vi "IRH1-2T_ConstructiveHeuristic.vi"(9 "Initial Construction Heursitic":T2, 10 "Scheduler":T1, 11 "Proocessing Times MxJ":u16[][](array[numeric])=[[1, 69, 192, 47, 292, 28, 166, 205], [146, 96, 177, 62, 37, 145, 3, 334], [99, 182, 133, 113, 9, 239, 27, 198], [159, 182, 132, 158, 183, 38, 142, 6], [92, 63, 114, 144, 180, 199, 136, 72], [119, 31, 9, 163, 139, 158, 350, 31], [46, 30, 59, 290, 156, 90, 175, 154], [338, 347, 184, 23, 4, 103, 1, 0]]) -> (1 "Due Dates":u16[](array[numeric]), 2 "Total Tardiness":u16, 3 "IRH2T Schedule Out":u16[](array[numeric]))   [LabVIEW 2013]
uses:
  Initial Construction Heuristic.ctl
  GA/Controls/Scheduler Type.ctl
  Classes/Scheduler_Class/Prins FIFO Scheduler Methods and Controls/Methods/UpdateMachineGaps.vi
  Classes/Scheduler_Class/Prins FIFO Scheduler Methods and Controls/Methods/UpdateJobGaps.vi
  Classes/Scheduler_Class/Prins FIFO Scheduler Methods and Controls/Methods/Find Intersecting Gaps.vi
  Classes/Scheduler_Class/Prins FIFO Scheduler Methods and Controls/Methods/Transform to Plain Job and Machine Gaps Array.vi
  Classes/Scheduler.lvclass
panel:
  in  "Proocessing Times (8x8)":u16[][](array[numeric])=[[1, 69, 192, 47, 292, 28, 166, 205], [146, 96, 177, 62, 37, 145, 3, 334], [99, 182, 133, 113, 9, 239, 27, 198], [159, 182, 132, 158, 183, 38, 142, 6], [92, 63, 114, 144, 180, 199, 136, 72], [119, 31, 9, 163, 139, 158, 350, 31], [46, 30, 59, 290, 156, 90, 175, 154], [338, 347, 184, 23, 4, 103, 1, 0]]
  out "Machine Completion Times":u16[](array[numeric])
  out "Completion Times":u16[][](array[numeric])
  out "Job Completion Times":i32[](array[numeric])
  out "String":string
  out "LPT Array":i32[](array[numeric])
  # "1, 69, 192, 47, 292, 28, 166, 205], \n[146, 96, 177, 62, 37, 145, 3, 334], \n[99, 182, 133, 113, 9, 239, 27, 198], \n[159, 182, 132, 158, 183, 38, 142, 6], \n[92, 63, 114, 144, 180, 199, 136, 72], \n[119, 31, 9, 163, 139, 158, 350, 31], \n[46, 30, 59, 290, 156, 90, 175, 154], \n[338, 347, 184, 23, 4, 103, 1, 0]]"
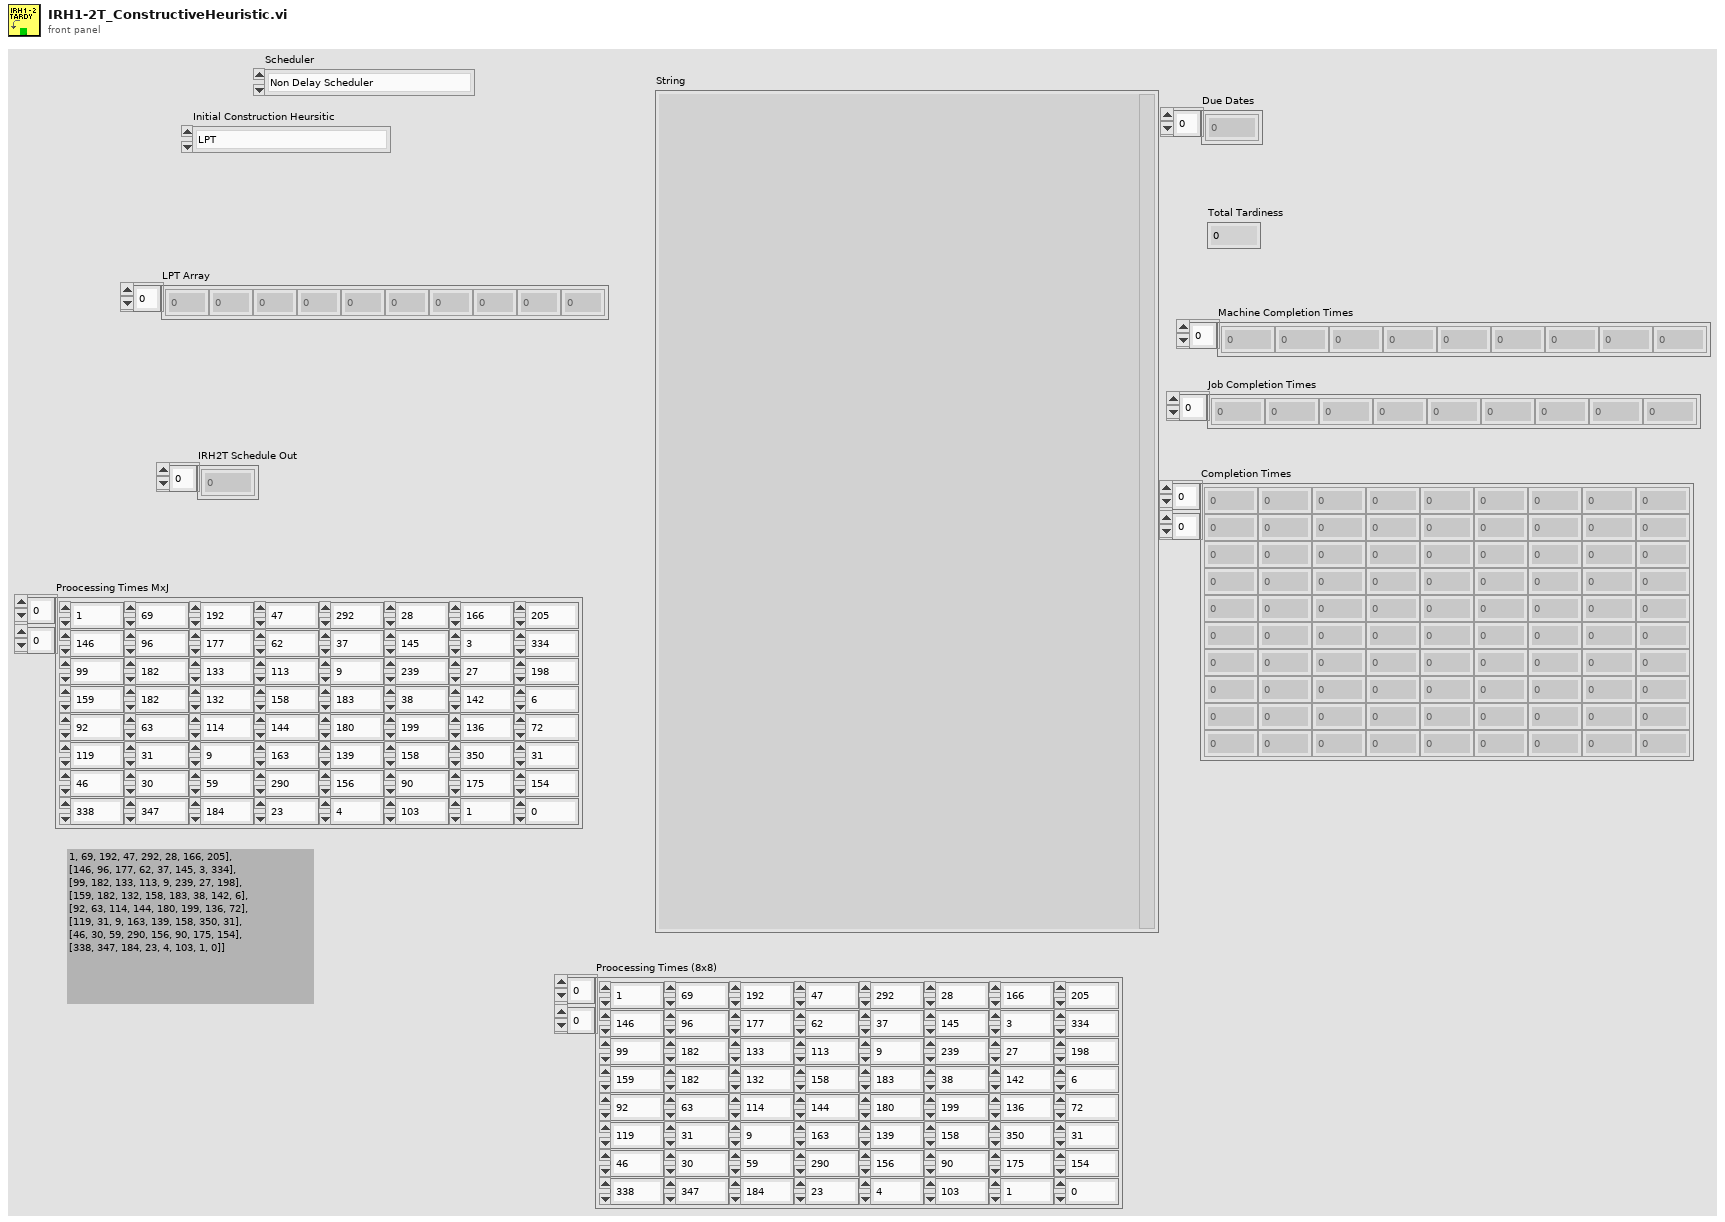
[diagram p1: front panel]
types:
  T1 = typedef "Scheduler Type.ctl" = enum16{"Non Delay Scheduler", "GT Active Scheduler", "My Faulty Scheduler", "Prins FIFO Scheduler", "SemiActive Scheduler", "Modified GT Scheduler"}
  T2 = typedef "Initial Construction Heuristic.ctl" = enum16{"LPT", "SPT", "EDD"}
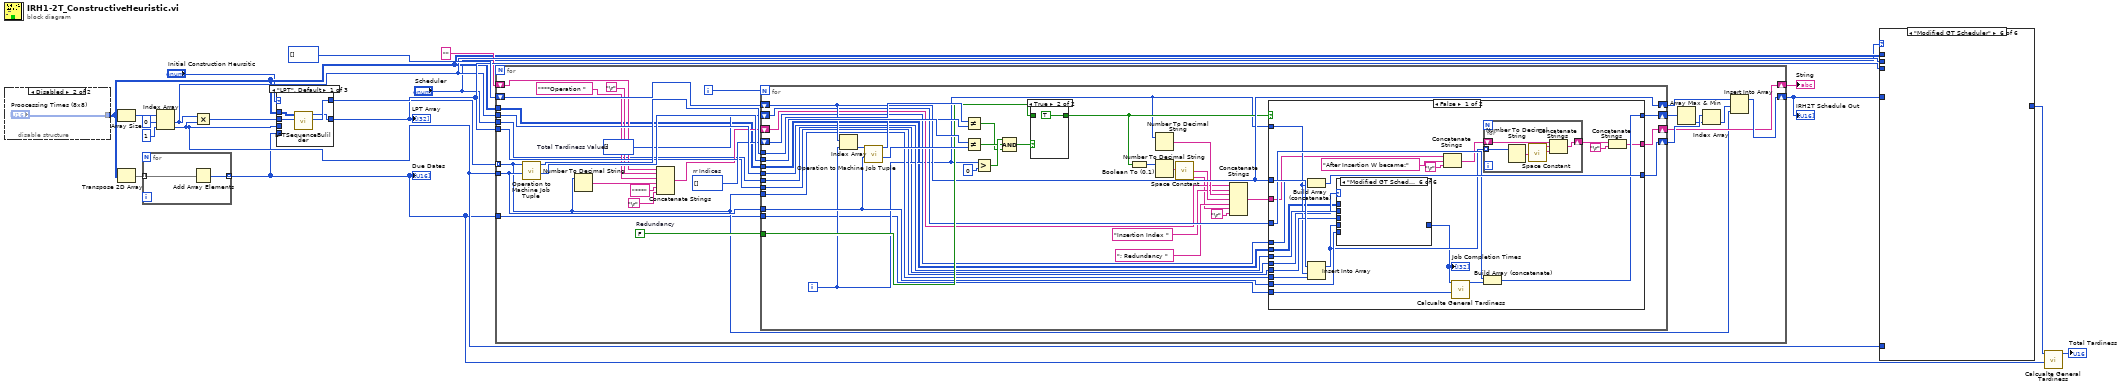
[diagram p0: block diagram]
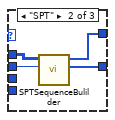
[diagram p2: hidden frame]
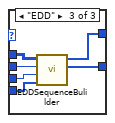
[diagram p3: hidden frame]
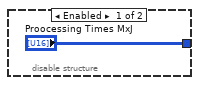
[diagram p4: hidden frame]
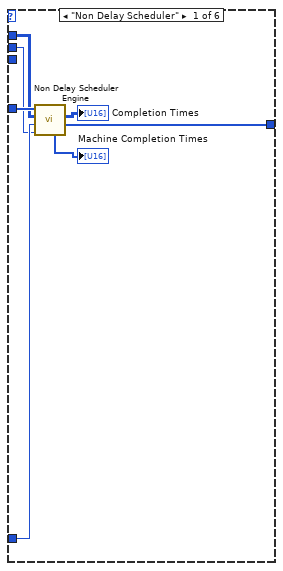
[diagram p5: hidden frame]
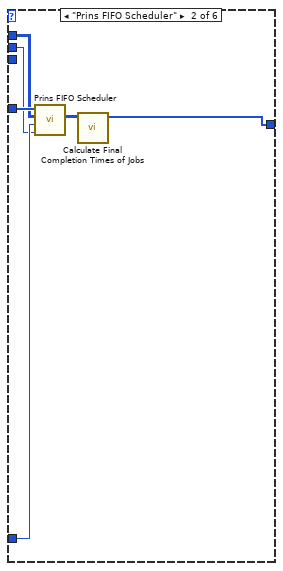
[diagram p6: hidden frame]
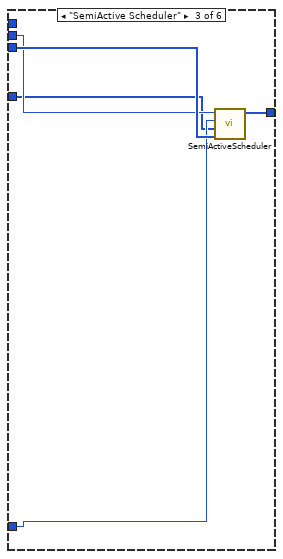
[diagram p7: hidden frame]
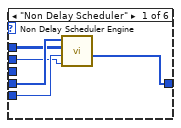
[diagram p10: hidden frame]
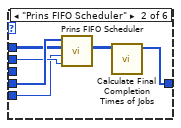
[diagram p11: hidden frame]
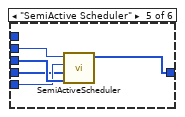
[diagram p14: hidden frame]
diagram:
  n1 = disable-structure shown="Disabled" {
    disable-tunnel: ["Proocessing Times MxJ" "Proocessing Times (8x8)"] -> w7
    frame Enabled {
    }
    frame Disabled {
    }
  }
  n2 = Array Size(array=w7) -> (size(s)=w19:i32[])
  n3 = Transpose 2D Array(2D array=w7) -> (transposed array=w10:u16[][])
  n4 = for {
    tunnel: w10 -> [w23] mode=indexing
    tunnel: [w22] -> w3 mode=indexing
    n5 = Add Array Elements(numeric array=w23) -> (sum=w22:u16)
  }
  "Due Dates" <- w3
  n6 = Index Array(array=w19, index #1=0 ("index"), index #2=1 ("index")) -> (element #1=w14:i32, element #2=w5:i32)
  n7 = Multiply(x=w14, y=w5) -> (x*y=w8:i32)
  n8 = case shown="\"LPT\", Default" "Initial Construction Heursitic" {
    tunnel: [w27 w29 w35] -> w15
    tunnel: [w26 w28 w34] -> w11
    tunnel: w8 -> [w25 w30 w36]
    tunnel: w7 -> [w24 w31 w37]
    tunnel: w3 -> [_ _ w32]
    tunnel: w5 -> [_ _ w33]
    frame "LPT", Default {
      n9 = call "LPTSequenceBulilder.vi"("Number Of Operations"=w25, "Proocessing Times MxJ"=w24) -> ("Falttened Processing Times"=w27:u16[], "LPT Sequence"=w26:i32[])  [unwired: 8 in]
    }
    frame "SPT" {
      n10 = call "SPTSequenceBulilder.vi"("Number Of Operations"=w30, "Proocessing Times MxJ"=w31) -> ("SPT Sequence"=w28:i32[], "Flattened Processing Times"=w29:u16[])  [unwired: 8 in]
    }
    frame "EDD" {
      n11 = call "EDDSequenceBulilder.vi"("Due Dates"=w32, "Number Of Machines"=w33, "Number Of Operations"=w36, "Proocessing Times MxJ"=w37) -> ("EDD Squence"=w34:i32[], "Flattened Processing Times"=w35:u16[])  [unwired: 6 in]
    }
  }
  "LPT Array" <- w11
  n12 = for {
    tunnel: w11 -> [w47] mode=indexing
    tunnel: w5 -> [w59]
    shift-right: [w51] -> w9
    shift-left: u16[] [] -> [w63]
    tunnel: w15 -> [w52]
    tunnel: w14 -> [w58]
    shift-right: [w49] -> w12
    shift-left: "" -> [w48]
    tunnel: w7 -> [w40]
    tunnel: "Scheduler" -> [w39]
    tunnel: w3 -> [w38]
    i -> [w65]
    w56 = i32[] []  # Total Tardiness Values
    w57 = i32[] []  # rr Indices
    w64 = FALSE  # Redundancy
    n13 = call "Operation to Machine Job Tuple.vi"("Number of Machines"=w59, "Operation Number"=w47) -> ("Job No"=w60:i32, "Machine No"=w61:i32)  [unwired: 8 in]
    n14 = Number To Decimal String(number=w47) -> (decimal integer string=w45:string)  [unwired: 1 in]
    n15 = Concatenate Strings(w48, "\r", "***Operation " ("string"), w45, "***" ("string"), "\r") -> (w44:string)
    n16 = for {
      N: w65 -> [_]
      shift-right: [w91] -> w62
      shift-left: w63 -> [w91]
      tunnel: w61 -> [w95]
      tunnel: w60 -> [w98]
      tunnel: w59 -> [w88]
      tunnel: w64 -> [w92]
      tunnel: w47 -> [w90]
      tunnel: w52 -> [w89]
      tunnel: w58 -> [w87]
      shift-right: [w85] -> w55
      shift-left: w57 -> [w86]
      shift-right: [w83] -> w50
      shift-left: w56 -> [w84]
      shift-right: [w81] -> w49
      shift-left: w44 -> [w75]
      tunnel: w40 -> [w68]
      tunnel: w39 -> [w67]
      tunnel: w38 -> [w66]
      i -> [w72]
      n17 = Index Array(array=w91, index=w72) -> (element=w80:u16)
      n18 = call "Operation to Machine Job Tuple.vi"("Number of Machines"=w88, "Operation Number"=w80) -> ("Job No"=w97:i32, "Machine No"=w94:i32)  [unwired: 8 in]
      n19 = Not Equal?(x=w95, y=w94) -> (x != y?=w82:bool)
      n20 = Not Equal?(x=w98, y=w97) -> (x != y?=w96:bool)
      n21 = Greater?(x=w72, y=0) -> (0:w99:bool)
      n22 = Compound Arithmetic op=AND(w99, w96, w82) -> (w93:bool)
      n23 = case shown="True" w93 {
        tunnel: w92 -> [w148 _]
        tunnel: [w148 TRUE ("Redundancy")] -> w73
        frame False {
        }
        frame True {
        }
      }
      n24 = Boolean To (0,1)(Boolean=w73) -> (0, 1=w71:i16)
      n25 = Number To Decimal String(number=w72) -> (decimal integer string=w77:string)  [unwired: 1 in]
      n26 = Number To Decimal String(number=w71) -> (decimal integer string=w70:string)  [unwired: 1 in]
      n27 = call <vilib>:"Space Constant.vi"() -> ("String"=w78:string)
      n28 = Concatenate Strings(w75, "Insertion Index " ("string"), w77, w78, "; Redundancy " ("string"), w70, "\r") -> (w74:string)
      n29 = case shown="False" w73 {
        tunnel: w91 -> [w123 _]
        tunnel: w90 -> [w122 _]
        tunnel: w89 -> [w121 _]
        tunnel: w88 -> [w120 _]
        tunnel: w87 -> [w119 _]
        tunnel: w86 -> [w118 w147]
        tunnel: w72 -> [w112 _]
        tunnel: [w117 w147] -> w85
        tunnel: w84 -> [w116 w146]
        tunnel: [w115 w146] -> w83
        tunnel: [w113 w145] -> w81
        tunnel: w74 -> [w111 w145]
        tunnel: w68 -> [w104 _]
        tunnel: w67 -> [w105 _]
        tunnel: w66 -> [w101 _]
        frame False {
          n30 = Build Array (concatenate)(w118, w112) -> (w117:i32[])
          n31 = Insert Into Array(array=w123, index=w112, new element=w122) -> (w114:u16[])
          n32 = case shown="\"Modified GT Scheduler\"" w105 {
            tunnel: w121 -> [_ _ _ _ w139 _]
            tunnel: w120 -> [w127 w129 _ _ w138 _]
            tunnel: w119 -> [w126 w130 _ _ w137 _]
            tunnel: [w125 w134 _ _ w136 _] -> w103
            tunnel: w114 -> [w128 w132 _ _ w135 _]
            tunnel: w104 -> [w124 w131 _ _ _ _]
            frame "Non Delay Scheduler" {
              n33 = call "Non Delay Scheduler Engine.vi"("Number of  Jobs"=w126, "Number of Machines"=w127, "Processing Times"=w124, "Schedule"=w128) -> ("Job Completion Times"=w125:u16[])  [unwired: 2 in, 5 out]
            }
            frame "Prins FIFO Scheduler" {
              n34 = call "Prins FIFO Scheduler.vi"("Number of Jobs"=w130, "Number of Machines"=w129, "Processing Times(MxJ)"=w131, "Schedule In"=w132) -> ("Completion Times (MxJ)"=w133:i32[][])  [unwired: 6 in, 1 out]
              n35 = call "Calculate Final Completion Times of Jobs.vi"("Completion Times (MxJ)"=w133) -> ("Job Completion Times"=w134:i32[])  [unwired: 10 in]
            }
            frame "GT Active Scheduler" {
            }
            frame "My Faulty Scheduler" {
            }
            frame "SemiActive Scheduler" {
              n36 = call "SemiActiveScheduler.vi"("Proocessing Times"=w139, "Schedule"=w135, "Number Of Machines"=w138, "Number Of Jobs"=w137) -> ("Job Completion Times"=w136:i32[])  [unwired: 5 in, 2 out]
            }
            frame "Modified GT Scheduler" {
            }
          }
          "Job Completion Times" <- w103
          n37 = Concatenate Strings(w111, "After Insertion W became:" ("string"), "\r") -> (w108:string)
          n38 = call "Calcualte General Tardiness.vi"("Due Dates"=w101, "Job Completion Times"=w103) -> ("Total Tardiness (U16)"=w102:u16)  [unwired: 9 in]
          n39 = for {
            tunnel: w114 -> [w144] mode=indexing
            shift-right: [w141] -> w107
            shift-left: w108 -> [w143]
            n40 = Number To Decimal String(number=w144) -> (decimal integer string=w142:string)  [unwired: 1 in]
            n41 = call <vilib>:"Space Constant.vi"() -> ("String"=w140:string)
            n42 = Concatenate Strings(w143, w142, w140) -> (w141:string)
          }
          n43 = Build Array (concatenate)(w116, w102) -> (w115:i32[])
          n44 = Concatenate Strings(w107, "\r") -> (w113:string)
        }
        frame True {
        }
      }
    }
    n45 = Array Max & Min(array=w50) -> (min index (indices)=w54:i32)  [unwired: 3 out]
    n46 = Index Array(array=w55, index=w54) -> (element=w53:i32)
    n47 = Insert Into Array(array=w62, index=w53, new element=w47) -> (w51:u16[])
  }
  "String" <- w12
  "IRH2T Schedule Out" <- w9
  n48 = case shown="\"Modified GT Scheduler\"" "Scheduler" {
    tunnel: w9 -> [w156 w162 w163 _ _ _]
    tunnel: w15 -> [_ _ w167 _ _ _]
    tunnel: w5 -> [w155 w160 w166 _ _ _]
    tunnel: w14 -> [w154 w159 w165 _ _ _]
    tunnel: [w153 w157 w164 _ _ _] -> w4
    tunnel: w7 -> [w150 w161 _ _ _ _]
    frame "Non Delay Scheduler" {
      n49 = call "Non Delay Scheduler Engine.vi"("Number of  Jobs"=w154, "Number of Machines"=w155, "Processing Times"=w150, "Schedule"=w156) -> ("Job Completion Times"=w153:u16[], "Completion Times"=→"Completion Times":u16[][], "Machine Completion Times"=→"Machine Completion Times":u16[])  [unwired: 2 in, 3 out]
    }
    frame "Prins FIFO Scheduler" {
      n50 = call "Prins FIFO Scheduler.vi"("Number of Jobs"=w159, "Number of Machines"=w160, "Processing Times(MxJ)"=w161, "Schedule In"=w162) -> ("Completion Times (MxJ)"=w158:i32[][])  [unwired: 6 in, 1 out]
      n51 = call "Calculate Final Completion Times of Jobs.vi"("Completion Times (MxJ)"=w158) -> ("Job Completion Times"=w157:i32[])  [unwired: 10 in]
    }
    frame "SemiActive Scheduler" {
      n52 = call "SemiActiveScheduler.vi"("Proocessing Times"=w167, "Schedule"=w163, "Number Of Machines"=w166, "Number Of Jobs"=w165) -> ("Job Completion Times"=w164:i32[])  [unwired: 5 in, 2 out]
    }
    frame "GT Active Scheduler" {
    }
    frame "My Faulty Scheduler" {
    }
    frame "Modified GT Scheduler" {
    }
  }
  n53 = call "Calcualte General Tardiness.vi"("Due Dates"=w3, "Job Completion Times"=w4) -> ("Total Tardiness (U16)"=→"Total Tardiness":u16)  [unwired: 9 in]
